vi "Config Get prop.vi"(10 "Signal Channel":u32, 11 "Attributes in":T1[](array[typedef])) -> (1 "Cancelled?":bool, 2 "Channel out":u32, 3 "Attributes out":T1[](array[typedef]))   [LabVIEW 2020, in "Get DDT Properties.lvlib"]
doc: "Retrieves the attributes of the dynamic data you wire to <B>Signals In</B>."
uses:
  <vilib>/express/express signal manip/GetorSetDDTAttributes/Get DDT Attributes/Get DDT Properties.lvlib
  <vilib>/express/express signal manip/GetorSetDDTAttributes/Shared VIs/Attributes data.ctl
  <vilib>/express/express signal manip/GetorSetDDTAttributes/Shared VIs/Input.ctl
  <vilib>/express/express signal manip/GetorSetDDTAttributes/Shared VIs/Attributes name.ctl
  <vilib>/express/express signal manip/GetorSetDDTAttributes/Get DDT Attributes/Get DDT Properties.xnode
  <vilib>/express/express signal manip/GetorSetDDTAttributes/Shared VIs/GetSetShared.lvlib
panel:
  in  "Signal Index":u32
  in  "Unit":bool
  in  "X dimension":bool
  in  "Timestamp":bool
  in  "Start timestamp":bool
  in  "Time mode":bool
  in  "Signal name":bool
  in  "help":bool
  in  "Cancel":bool
  in  "OK":bool
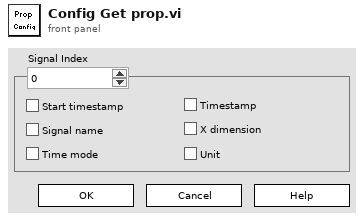
[diagram p1: front panel]
types:
  T1 = typedef "GetSetShared.lvlib/Attributes data.ctl" = cluster{"State":T2, "Attributes Name":T3, "Value":variant, "wired?":bool}
  T2 = typedef "GetSetShared.lvlib/Input.ctl" = bool
  T3 = typedef "GetSetShared.lvlib/Attributes name.ctl" = enum16{"NI_ChannelName", "NI_ExpIsRelativeTime", "NI_ExpTimeStamp", "NI_ExpStartTimeStamp", "NI_ExpXDimension", "NI_UnitDescription"}
  T4 = cluster{"Description":string, "Path":path, "Tag":string}
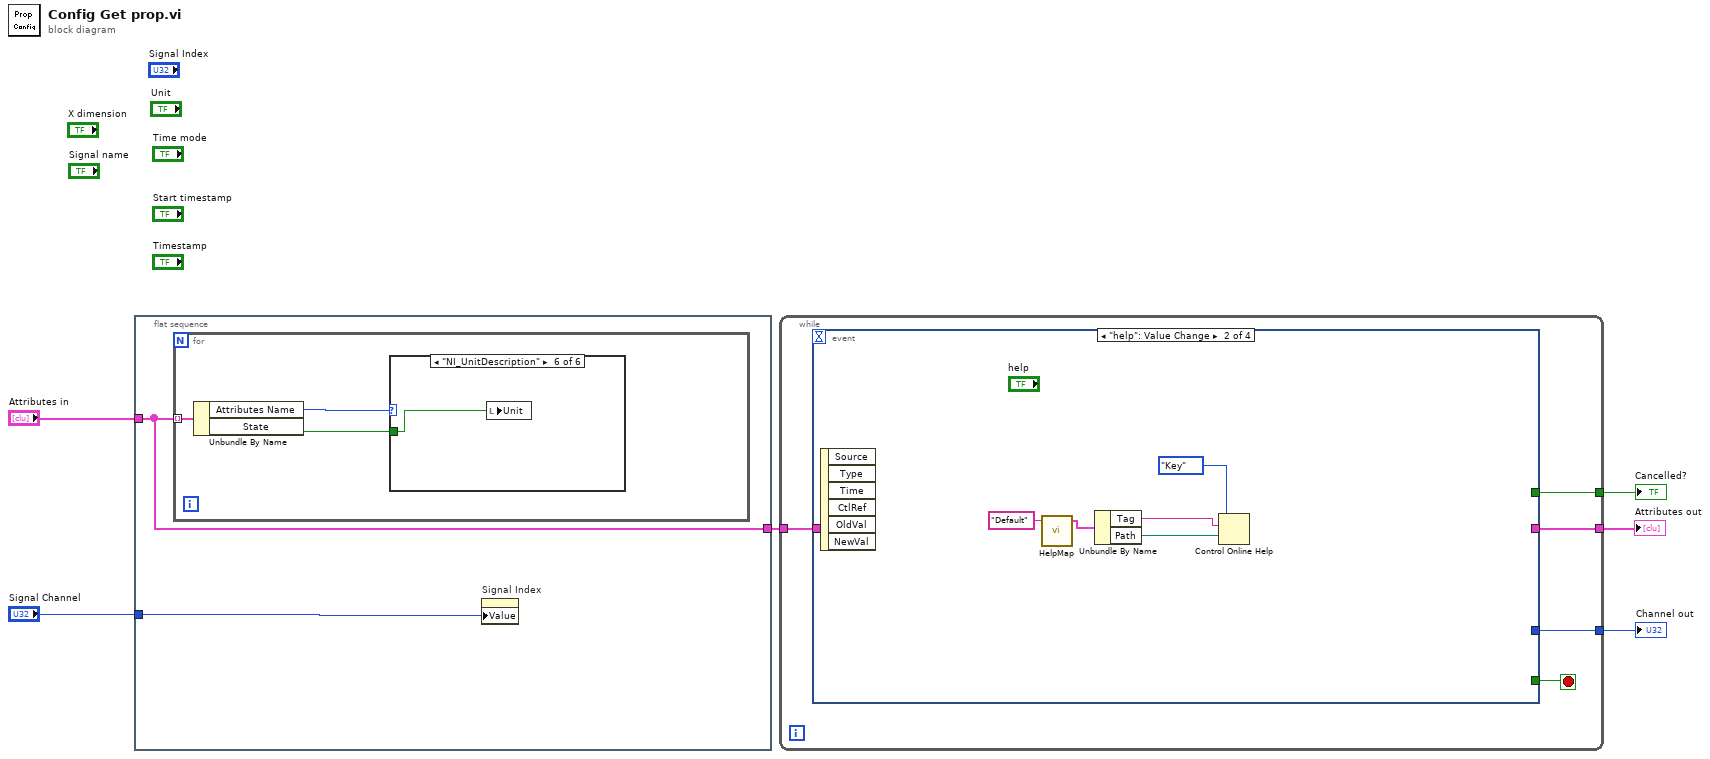
[diagram p0: block diagram]
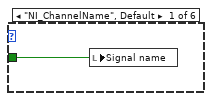
[diagram p2: hidden frame]
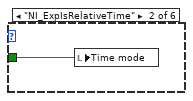
[diagram p3: hidden frame]
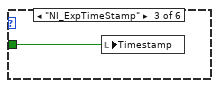
[diagram p4: hidden frame]
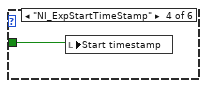
[diagram p5: hidden frame]
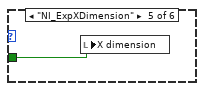
[diagram p6: hidden frame]
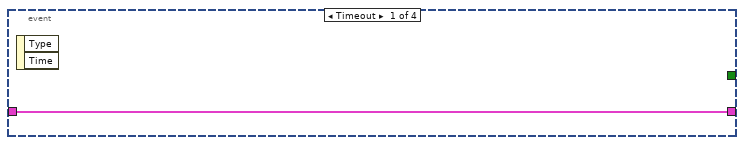
[diagram p7: hidden frame]
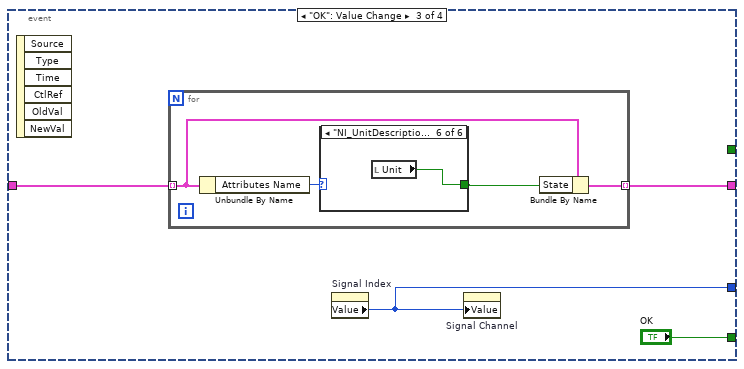
[diagram p8: hidden frame]
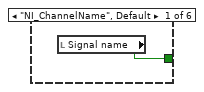
[diagram p9: hidden frame]
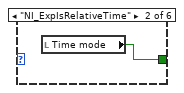
[diagram p10: hidden frame]
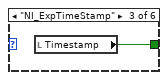
[diagram p11: hidden frame]
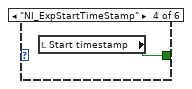
[diagram p12: hidden frame]
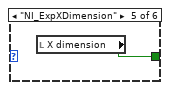
[diagram p13: hidden frame]
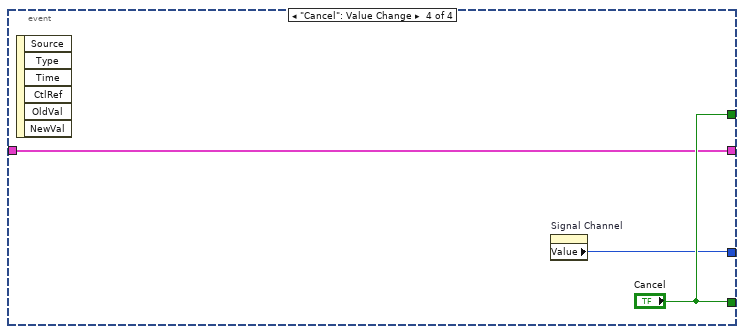
[diagram p14: hidden frame]
diagram:
  n1 = flat-sequence {
    tunnel: "Attributes in" -> [w8]
    tunnel: [w8] -> w4
    tunnel: "Signal Channel" -> [w7]
    frame #0 {
      n2 = for {
        tunnel: w8 -> [w11] mode=indexing
        n3 = Unbundle By Name(w11) -> ("Attributes Name"=w10:T3, "State"=w9:T2)
        n4 = case shown="\"NI_UnitDescription\"" w10 {
          tunnel: w9 -> [w12 w13 w14 w15 w16 w17]
          frame "NI_ChannelName", Default {
            n5 = local write "Signal name"(w12) -> ()
          }
          frame "NI_ExpIsRelativeTime" {
            n6 = local write "Time mode"(w13) -> ()
          }
          frame "NI_ExpTimeStamp" {
            n7 = local write "Timestamp"(w14) -> ()
          }
          frame "NI_ExpStartTimeStamp" {
            n8 = local write "Start timestamp"(w15) -> ()
          }
          frame "NI_ExpXDimension" {
            n9 = local write "X dimension"(w16) -> ()
          }
          frame "NI_UnitDescription" {
            n10 = local write "Unit"(w17) -> ()
          }
        }
      }
      n11 = property on="Signal Index" class="DigNum (strict)"("Value"=w7) -> ()  [unwired: 2 in, 2 out]
    }
  }
  n12 = while {
    tunnel: [w21] -> w6
    tunnel: w4 -> [w20]
    tunnel: [w19] -> w3
    tunnel: [w18] -> w2
    stop <- w22 stop-if-true
    n13 = event shown="[1] \"help\": Value Change" {
      selector: _ -> [_ _ _ _]
      dyn-events: _ -> [_ _ _ _]
      timeout: _ -> [_ _ _ _]
      tunnel: [_ _ "OK" "Cancel"] -> w22
      tunnel: [_ _ _ "Cancel"] -> w21
      tunnel: w20 -> [w23 _ w31 w44]
      tunnel: [w23 _ w30 w44] -> w19
      tunnel: [_ _ w29 w43] -> w18
      event Timeout {
        n14 = event-data() -> ()  [unwired: 3 out]
      }
      event "help": Value Change {
        n15 = event-data() -> ()  [unwired: 7 out]
        n16 = call <vilib>:"HelpMap.vi"("Standard Help ID"="Default") -> ("Standard Help Info"=w26:T4)  [unwired: 2 in, 2 out]
        n17 = Unbundle By Name(w26) -> ("Tag"=w25:string, "Path"=w24:path)
        n18 = Control Online Help(2:w24, 3:w25, 4:enum16{"Contents", "Key", "Close"}."Key" ("Operation")) -> ()  [unwired: 1 in, 1 out]
      }
      event "OK": Value Change {
        n19 = event-data() -> ()  [unwired: 7 out]
        n20 = for {
          tunnel: w31 -> [w35] mode=indexing
          tunnel: [w34] -> w30 mode=indexing
          n21 = Unbundle By Name(w35) -> ("Attributes Name"=w36:T3)
          n22 = case shown="\"NI_UnitDescription\"" w36 {
            tunnel: [w37 w38 w39 w40 w41 w42] -> w33
            frame "NI_ChannelName", Default {
              n23 = local read "Signal name"() -> (w37:bool)
            }
            frame "NI_ExpIsRelativeTime" {
              n24 = local read "Time mode"() -> (w38:bool)
            }
            frame "NI_ExpTimeStamp" {
              n25 = local read "Timestamp"() -> (w39:bool)
            }
            frame "NI_ExpStartTimeStamp" {
              n26 = local read "Start timestamp"() -> (w40:bool)
            }
            frame "NI_ExpXDimension" {
              n27 = local read "X dimension"() -> (w41:bool)
            }
            frame "NI_UnitDescription" {
              n28 = local read "Unit"() -> (w42:bool)
            }
          }
          n29 = Bundle By Name(cluster=w35, "State"=w33) -> (w34:T1)
        }
        n30 = property on="Signal Index" class="DigNum (strict)"() -> ("Value"=w29:u32)  [unwired: 2 in, 2 out]
        n31 = property on="Signal Channel" class="DigNum (strict)"("Value"=w29) -> ()  [unwired: 2 in, 2 out]
      }
      event "Cancel": Value Change {
        n32 = event-data() -> ()  [unwired: 7 out]
        n33 = property on="Signal Channel" class="DigNum (strict)"() -> ("Value"=w43:u32)  [unwired: 2 in, 2 out]
      }
    }
  }
  "Cancelled?" <- w6
  "Attributes out" <- w3
  "Channel out" <- w2
